vi "Dmux4Way.vi"(2 "in":bool, 4 "sel":bool[](array[boolean])) -> (6 "a":bool, 7 "b":bool, 9 "c":bool, 10 "d":bool)   [LabVIEW 2014]
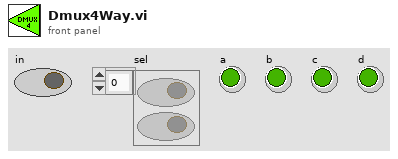
[diagram p1: front panel]
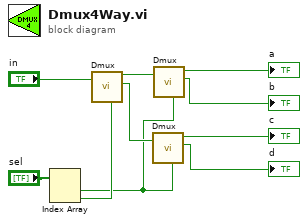
[diagram p0: block diagram]
diagram:
  n1 = Index Array(array="sel") -> (element #1=w1:bool, element #2=w8:bool)  [unwired: 2 in]
  n2 = call "Dmux.vi"("in"="in", "sel"=w8) -> ("a"=w7:bool, "b"=w6:bool)  [unwired: 4 in]
  n3 = call "Dmux.vi"("in"=w6, "sel"=w1) -> ("a"=→"c":bool, "b"=→"d":bool)  [unwired: 4 in]
  n4 = call "Dmux.vi"("in"=w7, "sel"=w1) -> ("a"=→"a":bool, "b"=→"b":bool)  [unwired: 4 in]
